vi "Append Error Details.vi"(8 "error in (no error)":errorcluster, 11 "Previous State and Argument(s)":string) -> (0 "error out":errorcluster)   [LabVIEW 2020]
doc: "Appends error details (State and Arguments) to error message.\n\nFor instructions on how to use the JKI State Machine, examples and video tutorials, visit:\nhttp://jkisoft.com/state-machine/"
panel:
  # "For instructions on how to use the JKI State Machine, examples and video tutorials, visit:\nhttp://jki.net/state-machine/\n\nJKI State Machine™\nhttp://jki.net/state-machine/\nCopyright (C) 2005-2024, JKI <info@jki.net>\nALL RIGHTS RESERVED"
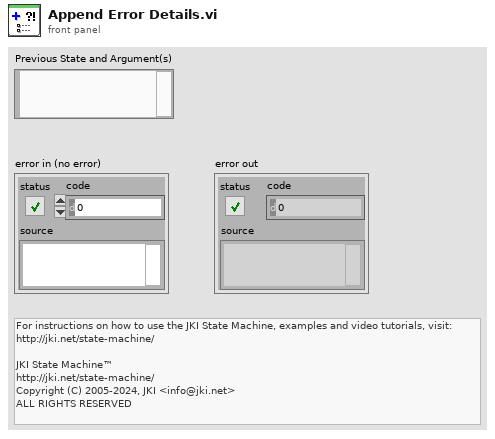
[diagram p1: front panel]
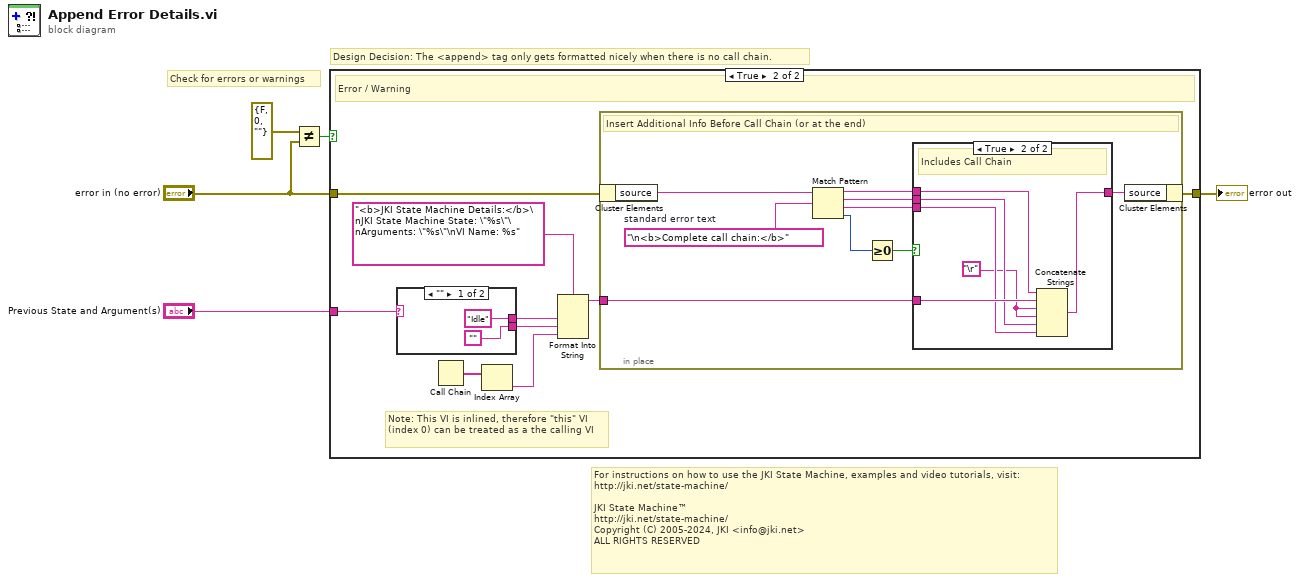
[diagram p0: block diagram]
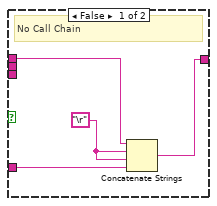
[diagram p3: hidden frame]
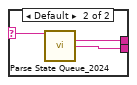
[diagram p4: hidden frame]
diagram:
  # "Check for errors or warnings"
  # "Design Decision: The <append> tag only gets formatted nicely when there is no call chain."
  # "For instructions on how to use the JKI State Machine, examples and video tutorials, visit:\nhttp://jki.net/state-machine/\n\nJKI State Machine™\nhttp://jki.net/state-machine/\nCopyright (C) 2005-2024, JKI <info@jki.net>\nALL RIGHTS RESERVED"
  n1 = Not Equal?(x=errorcluster {"status"=FALSE, "code"=0, "source"=""}, y="error in (no error)") -> (x != y?=w4:bool)
  n2 = case shown="True" w4 {
    tunnel: [w6 w7] -> w2
    tunnel: "error in (no error)" -> [w6 w9]
    tunnel: "Previous State and Argument(s)" -> [_ w10]
    frame False {
      # "NOT Error or Warning"
    }
    frame True {
      # "Note: This VI is inlined, therefore \"this\" VI (index 0) can be treated as a the calling VI"
      # "Error / Warning"
      n3 = case shown="\"\"" w10 {
        selector: w10 -> [_ w37]
        tunnel: ["Idle" ("Current State") w39] -> w12
        tunnel: ["" w38] -> w13
        frame "" {
        }
        frame Default {
          n4 = call "Parse State Queue_2024.vi"("State Queue"=w37) -> ("Current State"=w39:string, "Arguments"=w38:string)  [unwired: 12 in, 1 out]
        }
      }
      n5 = Call Chain() -> (call chain=w14:string[])
      n6 = Index Array(array=w14) -> (element=w15:string)  [unwired: 1 in]
      n7 = Format Into String(format string="<b>JKI State Machine Details:</b>\nJKI State Machine State: \"%s\"\nArguments: \"%s\"\nVI Name: %s" ("search string"), w12, w13, w15) -> (resulting string=w8:string)  [unwired: 2 in, 1 out]
      n8 = in-place {
        in-place-border: w8 -> [w23]
        w21 = "\n<b>Complete call chain:</b>"  # standard error text
        # "Insert Additional Info Before Call Chain (or at the end)"
        n9 = in-place-cluster #1(w9) -> ("source"=w22:string)
        n10 = Match Pattern(string=w22, regular expression=w21) -> (before substring=w18:string, match substring=w19:string, after substring=w20:string, offset past match=w17:i32)  [unwired: 1 in]
        n11 = Greater Or Equal To 0?(x=w17) -> (x >= 0?=w16:bool)
        n12 = case shown="True" w16 {
          tunnel: [w27 w34] -> w24
          tunnel: w23 -> [w25 w33]
          tunnel: w20 -> [_ w32]
          tunnel: w19 -> [_ w31]
          tunnel: w18 -> [w28 w30]
          frame False {
            w26 = "\r"
            # "No Call Chain"
            n13 = Concatenate Strings(w28, w26, w26, w25) -> (w27:string)
          }
          frame True {
            w29 = "\r"
            # "Includes Call Chain"
            n14 = Concatenate Strings(w30, w33, w29, w29, w31, w32) -> (w34:string)
          }
        }
        n15 = in-place-cluster #1("source"=w24) -> (w7:errorcluster)
      }
    }
  }
  "error out" <- w2
